vi "_Test_RDB Receive Points Core.vi"(10 "Data":u8[](array[numeric])) -> (3 "signal data":dbl[](array[numeric]) format="%.2f")   [LabVIEW 2023]
uses:
  <vilib>/xnet/xnet.llb/XNET Convert (Frame FlexRay to Signal).vi
  <vilib>/xnet/xnet.llb/XNET Create Session (Conversion).vi
  <vilib>/xnet/xnet.llb/XNET String To IO Name (Signal).vi
panel:
  out "Signals":refnum<k21>[](array[refnum])
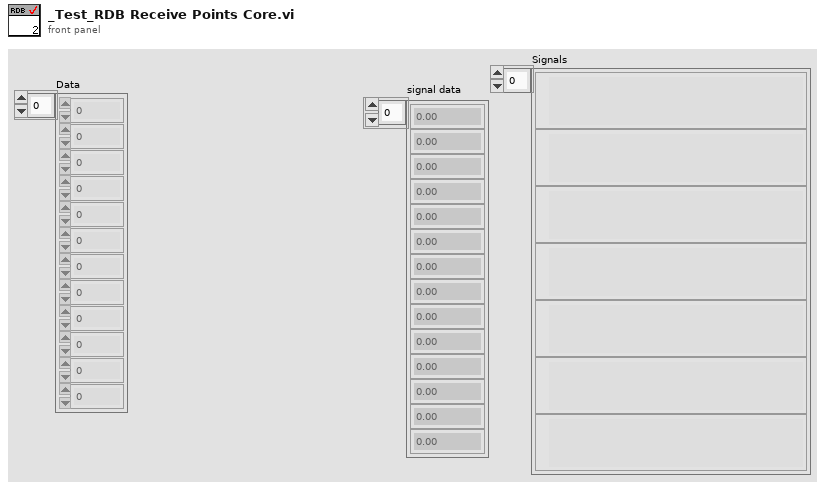
[diagram p1: front panel]
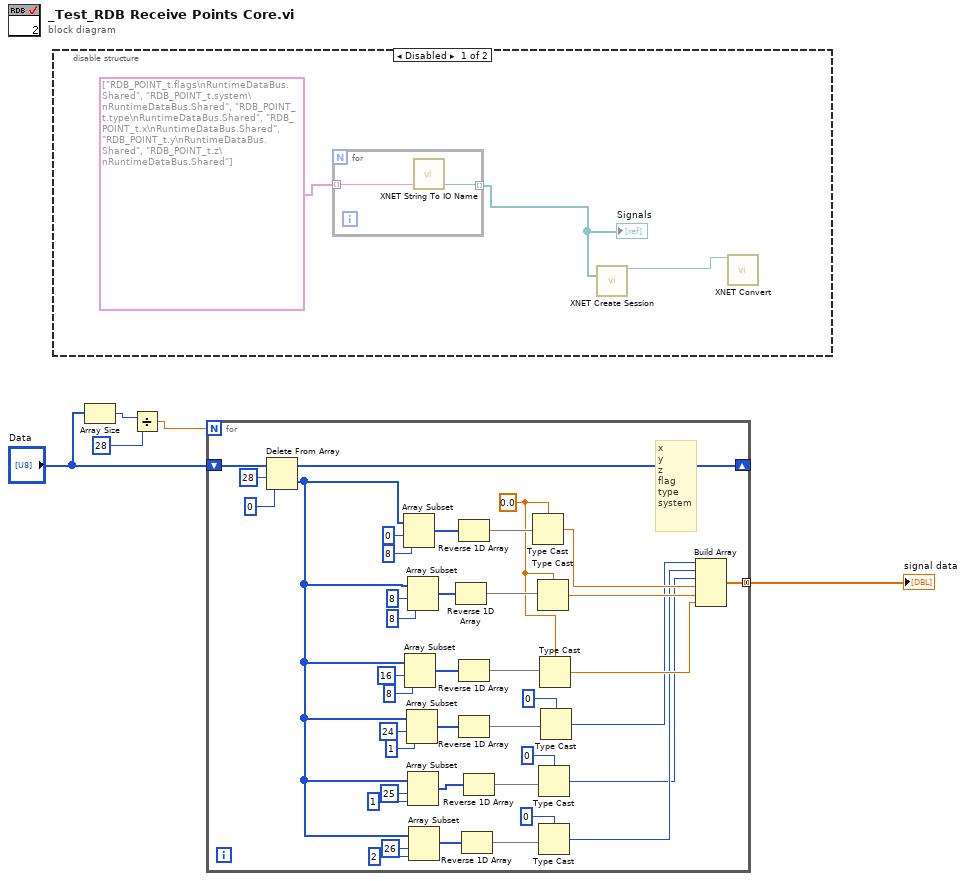
[diagram p0: block diagram]
diagram:
  n1 = disable-structure shown="Disabled" {
    frame Disabled {
      n2 = for {
        tunnel: string[] ["RDB_POINT_t.flags\nRuntimeDataBus.Shared", "RDB_POINT_t.system\nRuntimeDataBus.Shared", "RDB_POINT_t.type\nRuntimeDataBus.Shared", "RDB_POINT_t.x\nRuntimeDataBus.Shared", "RDB_POINT_t.y\nRuntimeDataBus.Shared", "RDB_POINT_t.z\nRuntimeDataBus.Shared"] -> [w10] mode=indexing
        tunnel: [w9] -> w7 mode=indexing
        n3 = call-poly <vilib>:"XNET String To IO Name.vi"("string"=w10) -> ("XNET Signal"=w9:refnum<k21>)  [unwired: 4 out]
      }
      "Signals" <- w7
      n4 = call-poly <vilib>:"XNET Create Session.vi"("signal list"=w7) -> ("session out"=w8:refnum<k21>)  [unwired: 13 in, 1 out]
      n5 = call-poly <vilib>:"XNET Convert.vi"("session in"=w8) -> ()  [unwired: 12 in, 3 out]
    }
    frame Enabled {
    }
  }
  n6 = Array Size(array="Data") -> (size(s)=w4:i32)
  n7 = Divide(x=w4, y=28) -> (x/y=w2:dbl)
  n8 = for {
    N: w2 -> [_]
    shift-right: [w47] -> _
    shift-left: "Data" -> [w50]
    tunnel: [w20] -> w1 mode=concatenating
    w21 = 0.0
    # "x\ny\nz\nflag\ntype\nsystem"
    n9 = Delete From Array(array=w50, length=28, index=0) -> (deleted portion=w40:u8[], array with subset deleted=w47:u8[])
    n10 = Array Subset(array=w40, index=0, length=8) -> (w45:u8[])
    n11 = Array Subset(array=w40, index=16, length=8) -> (w30:u8[])
    n12 = Array Subset(array=w40, index=24, length=1) -> (w29:u8[])
    n13 = Array Subset(array=w40, index=8, length=8) -> (w31:u8[])
    n14 = Array Subset(array=w40, index=25, length=1) -> (w28:u8[])
    n15 = Array Subset(array=w40, index=26, length=2) -> (w27:u8[])
    n16 = Reverse 1D Array(array=w31) -> (reversed array=w26:u8[])
    n17 = Reverse 1D Array(array=w45) -> (reversed array=w44:u8[])
    n18 = Reverse 1D Array(array=w30) -> (reversed array=w25:u8[])
    n19 = Reverse 1D Array(array=w29) -> (reversed array=w24:u8[])
    n20 = Reverse 1D Array(array=w27) -> (reversed array=w22:u8[])
    n21 = Reverse 1D Array(array=w28) -> (reversed array=w23:u8[])
    n22 = Type Cast(type=w21, x=w44) -> (*(type *) &x=w16:dbl)
    n23 = Type Cast(type=w21, x=w26) -> (*(type *) &x=w15:dbl)
    n24 = Type Cast(type=u8 0, x=w23) -> (*(type *) &x=w11:u8)
    n25 = Type Cast(type=u16 0, x=w22) -> (*(type *) &x=w12:u16)
    n26 = Type Cast(type=w21, x=w25) -> (*(type *) &x=w14:dbl)
    n27 = Type Cast(type=u8 0, x=w24) -> (*(type *) &x=w13:u8)
    n28 = Build Array(w13, w12, w11, w16, w15, w14) -> (w20:dbl[])
  }
  "signal data" <- w1
